vi "UpdateExpInfo.vi"(11 "File Paths":T1={"Local Save Path"=path "\\\\smbhome.uscs.susx.ac.uk\\cv222/Desktop/data", "Newton Save Path"=path "Z:/#Projects/Entanglement/data", "File Name"="test", "LocalSave"=TRUE}) -> (3 "ExpNum string":string)   [LabVIEW 2017]
uses:
  FilePaths.ctl
  GlobalExp.vi
  Global.lvlib
panel:
  in  "Array":cluster{"ExpNum":i16, "ExpType":string}[](array[cluster]) {"ExpNum" format="%_3f"}
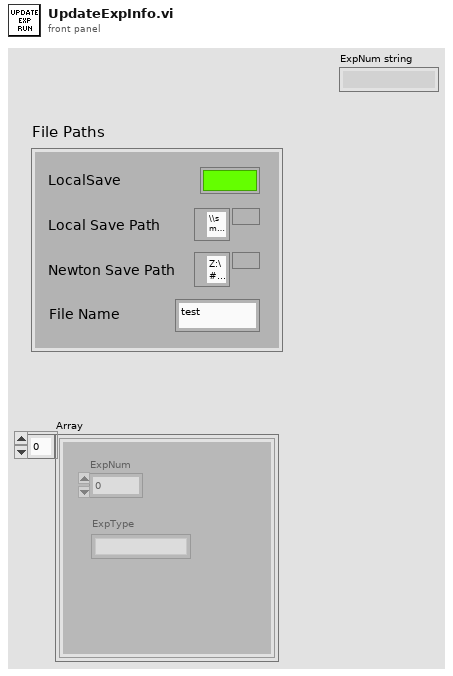
[diagram p1: front panel]
types:
  T1 = typedef "FilePaths.ctl" = cluster{"Local Save Path":path, "Newton Save Path":path, "File Name":string, "LocalSave":bool}
  T2 = enum16{"open", "replace", "create", "open or create", "replace or create", "replace or create with confirmation"}
  T3 = typedef "MasterExpControl.ctl" = cluster{"Main Steps":dbl, "Main Runs":dbl, "ExpStatus":enum16{"Innit", "Stop", "Idle", "MainRunning", "AuxRunning"}, "Main Current Step":dbl, "ExpNum":dbl, "NewData":bool, "date":string, "command":string, "Stop":bool, "Pause":bool, "Mathematica":string, "Main/Meta":bool, "UpdateMath":bool, "Camera":bool}
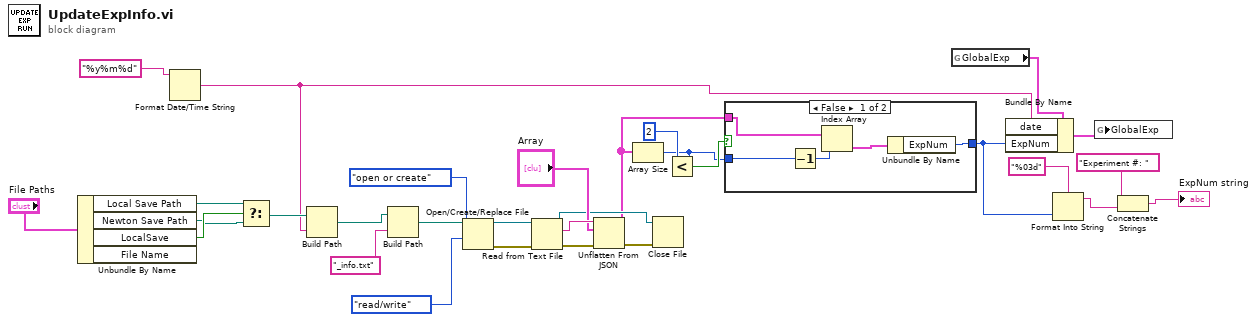
[diagram p0: block diagram]
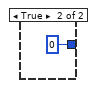
[diagram p2: hidden frame]
diagram:
  n1 = Unbundle By Name("File Paths") -> ("Local Save Path"=w25:path, "Newton Save Path"=w24:path, "LocalSave"=w26:bool)  [unwired: 1 out]
  n2 = Format Date/Time String(time format string (%c)="%y%m%d") -> (date/time string=w22:string)  [unwired: 2 in]
  n3 = Select(t=w25, s=w26, f=w24) -> (s? t:f=w23:path)
  n4 = Build Path(base path=w23, name or relative path=w22) -> (appended path=w21:path)
  n5 = Build Path(base path=w21, name or relative path="_info.txt") -> (appended path=w19:path)
  n6 = Open/Create/Replace File(file path (use dialog)=w19, operation (0:open)=T2."open or create", access (0:read/write)=enum16{"read/write", "read-only", "write-only"}."read/write") -> (refnum out=w15:refnum<file>, error out=w16:errorcluster)  [unwired: 3 in, 1 out]
  n7 = Read from Text File(file (use dialog)=w15, error in=w16) -> (refnum out=w10:refnum<file>, text=w13:string, error out=w14:errorcluster)  [unwired: 2 in, 1 out]
  n8 = Unflatten From JSON(JSON string=w13, type and defaults="Array", error in (no error)=w14) -> (value=w6:cluster{"ExpNum":i16, "ExpType":string}[], error out=w11:errorcluster)  [unwired: 4 in]
  n9 = Array Size(array=w6) -> (size(s)=w7:i32)
  n10 = Close File(refnum=w10, error in=w11) -> ()  [unwired: 2 out]
  n11 = Less?(x=w7, y=2) -> (x < y?=w9:bool)
  n12 = case shown="False" w9 {
    tunnel: [w33 i16 0 ("ExpNum")] -> w5
    tunnel: w7 -> [w32 _]
    tunnel: w6 -> [w31 _]
    frame False {
      n13 = Decrement(x=w32) -> (x-1=w35:i32)
      n14 = Index Array(array=w31, index=w35) -> (element=w34:cluster{"ExpNum":i16, "ExpType":string})
      n15 = Unbundle By Name(w34) -> ("ExpNum"=w33:i16)
    }
    frame True {
    }
  }
  n16 = global read "GlobalExp.vi" "GlobalExp"() -> (w29:T3)
  n17 = Bundle By Name(cluster=w29, "date"=w22, "ExpNum"=w5) -> (w28:T3)
  n18 = Format Into String(format string="%03d", w5) -> (resulting string=w2:string)  [unwired: 2 in, 1 out]
  n19 = global write "GlobalExp.vi" "GlobalExp"(w28) -> ()
  n20 = Concatenate Strings("Experiment #: " ("string"), w2) -> (→"ExpNum string":string)
